vi "Process CAN State.vi"(8 "error in (no error)":errorcluster, 11 "State":T1 {"fault code" format="%08x"; "last error" items=["None", "Stuff", "Form", "Ack", "Bit1", "Bit0", "CRC"]; "communication state" items=["Error Active", "Error Passive", "Bus Off", "Init"]}) -> (0 "error out":errorcluster, 3 "State":string)   [LabVIEW 2019, in "CAN Streaming Support Workspace Shared.lvlib"]
uses:
  CAN Streaming Support Workspace Shared.lvlib
  <vilib>/xnet/xnet.llb/XNET CAN Comm.ctl
  <vilib>/xnet/xnet.llb/XNET CAN Comm State.ctl
  <vilib>/xnet/xnet.llb/XNET CAN Last Err.ctl
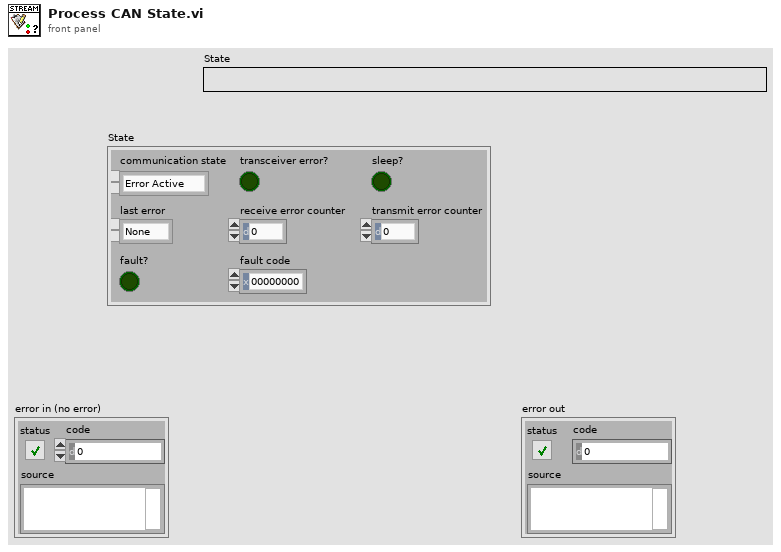
[diagram p1: front panel]
types:
  T1 = typedef "XNET CAN Comm.ctl" = cluster{"fault code":i32, "fault?":bool, "communication state":T2, "last error":T3, "receive error counter":u8, "transmit error counter":u8, "transceiver error?":bool, "sleep?":bool}
  T2 = typedef "XNET CAN Comm State.ctl" = u8
  T3 = typedef "XNET CAN Last Err.ctl" = u8
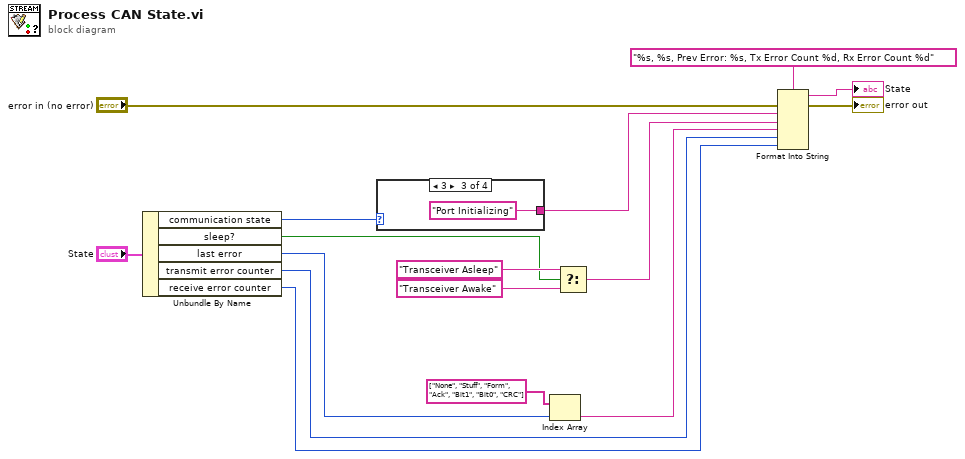
[diagram p0: block diagram]
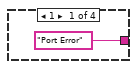
[diagram p2: hidden frame]
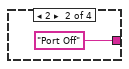
[diagram p3: hidden frame]
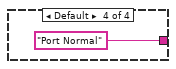
[diagram p4: hidden frame]
diagram:
  n1 = Unbundle By Name("State") -> ("communication state"=w6:T2, "sleep?"=w7:bool, "last error"=w3:T3, "transmit error counter"=w12:u8, "receive error counter"=w13:u8)
  n2 = case shown="3" w6 {
    tunnel: ["Port Error" "Port Off" "Port Initializing" "Port Normal"] -> w11
    frame 1 {
    }
    frame 2 {
    }
    frame 3 {
    }
    frame Default {
    }
  }
  n3 = Index Array(array=string[] ["None", "Stuff", "Form", "Ack", "Bit1", "Bit0", "CRC"] ("Strings []"), index=w3) -> (element=w2:string)
  n4 = Select(t="Transceiver Asleep", s=w7, f="Transceiver Awake") -> (s? t:f=w1:string)
  n5 = Format Into String(format string="%s, %s, Prev Error: %s, Tx Error Count %d, Rx Error Count %d", error in="error in (no error)", w11, w1, w2, w12, w13) -> (resulting string=→"State":string, error out=→"error out":errorcluster)  [unwired: 1 in]
